vi "NML GPIB Tester_ForEdwards.vi"(5 "?":string, 7 "Read":bool, 8 "Write":bool, 9 "VISA resource name":refnum<visa-resource-name>) -> (0 "error out":errorcluster, 4 "?":string)   [LabVIEW 2020]
doc: "General LabView-GPIB VI which allows the selection of a message termination mode, timeout and usefule english error codes and status messages.\nScott Hannahs, FBNML, Feb 1993"
panel:
  in  "Timeout (sec)":ext=1.0
  out "ÆTime":u32
  in  "Read Mode":u32(slide)=1 scale=0.0..2.0
  in  "Write Mode":u32(slide) scale=0.0..5.0
  in  "Clear REN\nwhen done":bool=TRUE
  out "Write Status":string
  out "Read Status":string
  in  "Byte count":u32=2000
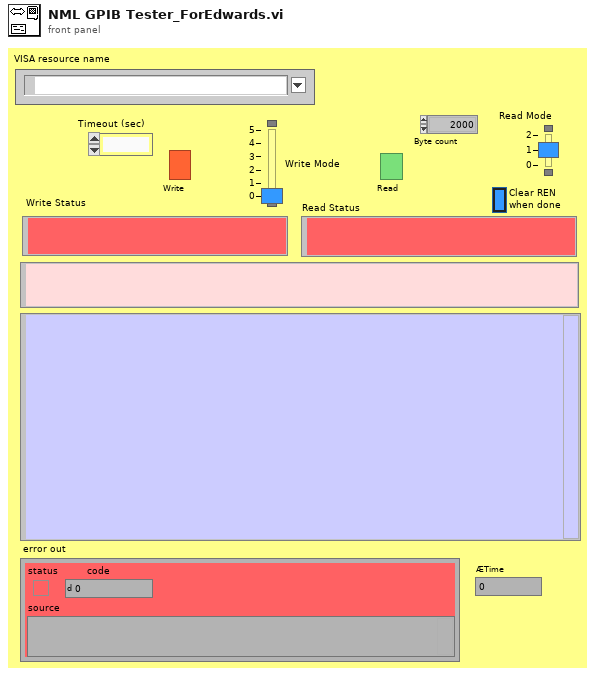
[diagram p1: front panel]
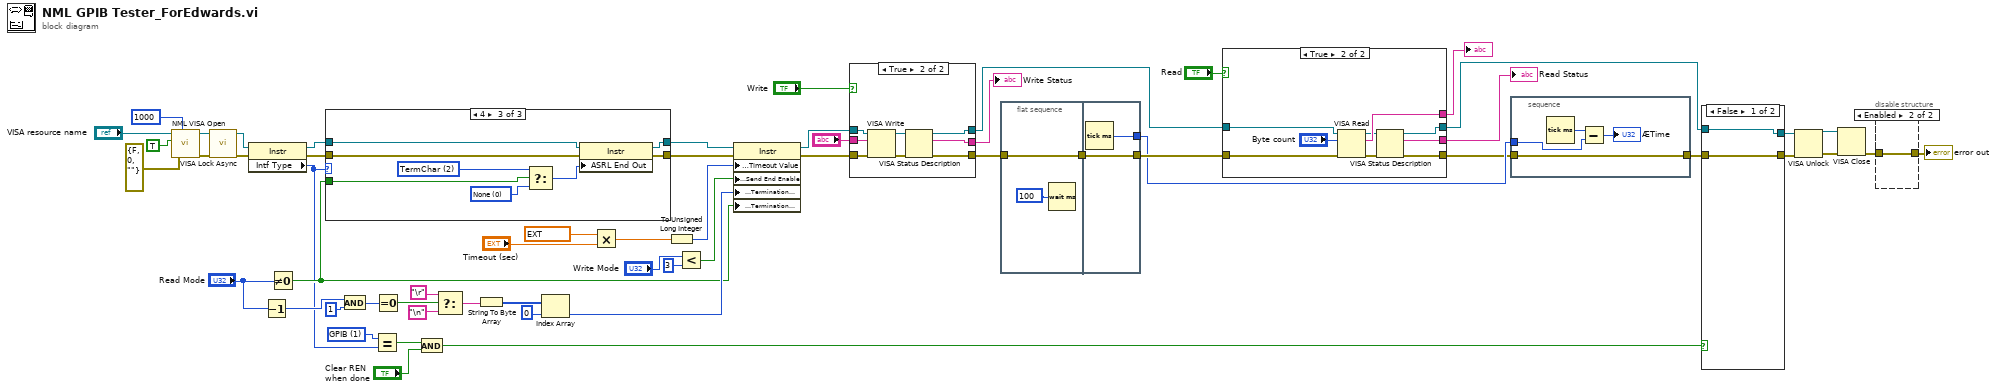
[diagram p0: block diagram]
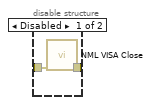
[diagram p2: hidden frame]
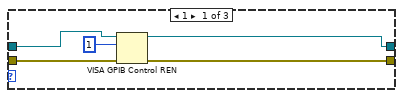
[diagram p3: hidden frame]
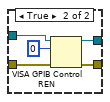
[diagram p5: hidden frame]
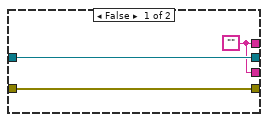
[diagram p6: hidden frame]
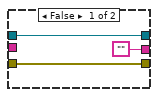
[diagram p7: hidden frame]
diagram:
  w7 = u16 1 items=["GPIB"=1, "VXI"=2, "GPIB-VXI"=3, "Serial"=4, "PXI"=5, "TCPIP"=6, "USB"=7, "FireWire"=9] ("Interface Information:Interface Type")
  n1 = call "NML VISA Open.vi"("VISA Open timeout (0)"=u32 1000 ("timeout (0)"), "error in (no error)"=errorcluster {"status"=FALSE, "code"=0, "source"=""}, "duplicate session (T)"=TRUE ("duplicate session (F)"), "VISA resource name"="VISA resource name") -> ("error out"=w15:errorcluster, "VISA resource name out"=w20:refnum<visa-resource-name>)  [unwired: 6 in]
  n2 = call <vilib>:"VISA Lock Async.vi"("error in (no error)"=w15, "VISA resource name"=w20) -> ("error out"=w14:errorcluster, "VISA resource name out"=w16:refnum<visa-resource-name>)  [unwired: 7 in, 1 out]
  n3 = property class="Instr"(reference=w16, error in=w14) -> (reference out=w18:refnum<visa-resource-name>, error out=w19:errorcluster, "Intf Type"=w8:u16)
  n4 = Decrement(x="Read Mode") -> (x-1=w38:u32)
  n5 = Not Equal To 0?(x="Read Mode") -> (x != 0?=w10:bool)
  n6 = case shown="4" w8 {
    tunnel: [w61 w64 w70] -> w22
    tunnel: [w60 w63 w69] -> w21
    tunnel: w19 -> [w59 w63 w71]
    tunnel: w18 -> [w58 w64 w72]
    tunnel: w10 -> [_ _ w66]
    frame 1 {
      n7 = VISA GPIB Control REN(8:w59, 10:u16 1 ("mode"), 11:w58) -> (0:w60:errorcluster, 3:w61:refnum<visa-resource-name>)
    }
    frame Default {
    }
    frame 4 {
      w65 = u16 2 items=["None", "Last Bit", "TermChar", "Break"] ("Serial Settings:End Mode for Writes")
      w67 = u16 0 items=["None", "Last Bit", "TermChar", "Break"] ("Serial Settings:End Mode for Writes")
      n8 = Select(t=w65, s=w66, f=w67) -> (s? t:f=w68:u16)
      n9 = property class="Instr"(reference=w72, error in=w71, "ASRL End Out"=w68) -> (reference out=w70:refnum<visa-resource-name>, error out=w69:errorcluster)
    }
  }
  n10 = And(x=w38, y=u32 1) -> (x .and. y?=w40:u32)
  n11 = Equal?(x=w7, y=w8) -> (x = y?=w6:bool)
  n12 = Equal To 0?(x=w40) -> (x = 0?=w41:bool)
  n13 = And(x=w6, y="Clear REN\nwhen done") -> (x .and. y?=w4:bool)
  n14 = Select(t="\r", s=w41, f="\n") -> (s? t:f=w36:string)
  n15 = String To Byte Array(string=w36) -> (unsigned byte array=w35:u8[])
  n16 = Index Array(array=w35, index=0 ("Index")) -> (element=w30:u8)
  n17 = Multiply(x=ext 1000.0, y="Timeout (sec)") -> (x*y=w56:ext)
  n18 = To Unsigned Long Integer(number=w56) -> (unsigned 32bit integer=w50:u32)
  n19 = Less?(x="Write Mode", y=u32 3) -> (x < y?=w45:bool)
  n20 = property class="Instr"(reference=w22, error in=w21, "General Settings:Timeout Value"=w50, "Message Based Settings:Send End Enable"=w45, "Message Based Settings:Termination Character"=w30, "Message Based Settings:Termination Character Enable"=w10) -> (reference out=w48:refnum<visa-resource-name>, error out=w49:errorcluster)
  n21 = case shown="True" "Write" {
    tunnel: w48 -> [w75 w83]
    tunnel: w49 -> [w74 w82]
    tunnel: [w75 w80] -> w53
    tunnel: [w74 w78] -> w28
    tunnel: ["" w77] -> w33
    tunnel: "?" -> [_ w76]
    frame False {
    }
    frame True {
      n22 = VISA Write(VISA resource name=w83, write buffer=w76, error in (no error)=w82) -> (VISA resource name out=w81:refnum<visa-resource-name>, error out=w79:errorcluster)  [unwired: 1 out]
      n23 = VISA Status Description(8:w79, 11:w81) -> (0:w78:errorcluster, 2:w77:string, 3:w80:refnum<visa-resource-name>)
    }
  }
  "Write Status" <- w33
  n24 = flat-sequence {
    tunnel: w28 -> [w85]
    tunnel: [w85] -> w3
    tunnel: w3 -> [w86]
    tunnel: [w86] -> w27
    tunnel: [w87] -> w25
    frame #0 {
      n25 = Wait (ms)(milliseconds to wait=u32 100) -> ()  [unwired: 1 out]
    }
    frame #1 {
      n26 = Tick Count (ms)() -> (millisecond timer value=w87:u32)
    }
  }
  n27 = case shown="True" "Read" {
    tunnel: w53 -> [w89 w96]
    tunnel: w27 -> [w90 w97]
    tunnel: [w90 w94] -> w24
    tunnel: [w89 w93] -> w31
    tunnel: [w88 w99] -> w51
    tunnel: [w88 w91] -> w29
    frame False {
      w88 = ""
    }
    frame True {
      n28 = VISA Read(VISA resource name=w96, byte count="Byte count", error in (no error)=w97) -> (VISA resource name out=w92:refnum<visa-resource-name>, read buffer=w99:string, error out=w95:errorcluster)  [unwired: 1 out]
      n29 = VISA Status Description(8:w95, 11:w92) -> (0:w94:errorcluster, 2:w91:string, 3:w93:refnum<visa-resource-name>)
    }
  }
  "?" <- w51
  "Read Status" <- w29
  n30 = stacked-sequence {
    tunnel: w24 -> [w103]
    tunnel: [w103] -> w26
    tunnel: w25 -> [w100]
    frame #0 {
      n31 = Tick Count (ms)() -> (millisecond timer value=w102:u32)
      n32 = Subtract(x=w102, y=w100) -> (x-y=→"ÆTime":u32)
    }
  }
  n33 = case shown="False" w4 {
    tunnel: w26 -> [w105 w110]
    tunnel: [w105 w109] -> w12
    tunnel: [w104 w108] -> w32
    tunnel: w31 -> [w104 w107]
    frame False {
    }
    frame True {
      n34 = VISA GPIB Control REN(8:w110, 10:u16 0 ("mode"), 11:w107) -> (0:w109:errorcluster, 3:w108:refnum<visa-resource-name>)
    }
  }
  n35 = VISA Unlock(8:w12, 11:w32) -> (0:w11:errorcluster, 3:w13:refnum<visa-resource-name>)
  n36 = VISA Close(VISA resource name=w13) -> ()  [unwired: 1 in, 1 out]
  n37 = disable-structure shown="Enabled" {
    disable-tunnel: [w112 w113] -> w47
    disable-tunnel: w11 -> [w111 w113]
    frame Disabled {
      n38 = call "NML VISA Close.vi"("Error In"=w111) -> ("Error Out"=w112:errorcluster)  [unwired: 10 in]
    }
    frame Enabled {
    }
  }
  "error out" <- w47
